vi "Butterfly_PullUp VPI VRL with Capacitance 20220628.vi"(0 "Semiconductor Module Context":T2, 3 "C_TH_Delta":dbl=0.03 format="%#_13g", 4 "VNAs Measurement Parameters":T1, 5 "error in (no error)":errorcluster, 9 "Start_v":dbl=10.0 format="%#_13g", 11 "Stop_v":dbl=41.0 format="%#_13g") -> (14 "Semiconductor Module Context Out":T2, 19 "error out":errorcluster)   [LabVIEW 2013]
uses:
  <vilib>/NI_TestStand_SemiconductorModule/NI_TestStand_Semiconductor_Module.lvlibp/PinMap/General/SemiconductorModuleContext.ctl
  VNA/VNAs Measurement Parameters.ctl
  <instrlib>/niDCPower/nidcpower.llb/niDCPower Wait For Event - Event.ctl
  <vilib>/NI_TestStand_SemiconductorModule/NI_TestStand_Semiconductor_Module.lvlibp/PinMap/General/Publish/PublishDataDouble2D.vi
  <vilib>/NI_TestStand_SemiconductorModule/NI_TestStand_Semiconductor_Module.lvlibp
  VNA/Pin Map API/VNA Custom Instrument.lvlib
panel:
  out "Site":i32
  out "RL Step":i32
  out "PI Step":i32
  out "C_TH_PU":dbl format="%#_3g"
  out "C_Free":dbl[](array[numeric]) format="%#_3g"
  out "max index":i32
  out "BF C PI":dbl format="%#_3g"
  out "C_VPI":dbl
  out "BF C RL":dbl format="%#_3g"
  out "C_VRL":dbl
  out "appended array":dbl[][](array[numeric]) format="%#_3g"
  out "S3 steps":dbl[](array[numeric]) format="%#_3g"
  out "S2 steps":dbl[](array[numeric]) format="%#_3g"
  out "S1 steps":dbl[](array[numeric]) format="%#_3g"
  out "S0 steps":dbl[](array[numeric]) format="%#_3g"
  out "BF values":dbl[](array[numeric])
  out "VRLs":dbl[](array[numeric])
  out "VPIs":dbl[](array[numeric])
  out "Multisite Cap Data":dbl[][][](array[numeric])
  out "BF Names":string[](array[string])
  out "BFSamples":i32
  in  "Step_v":dbl=1.0
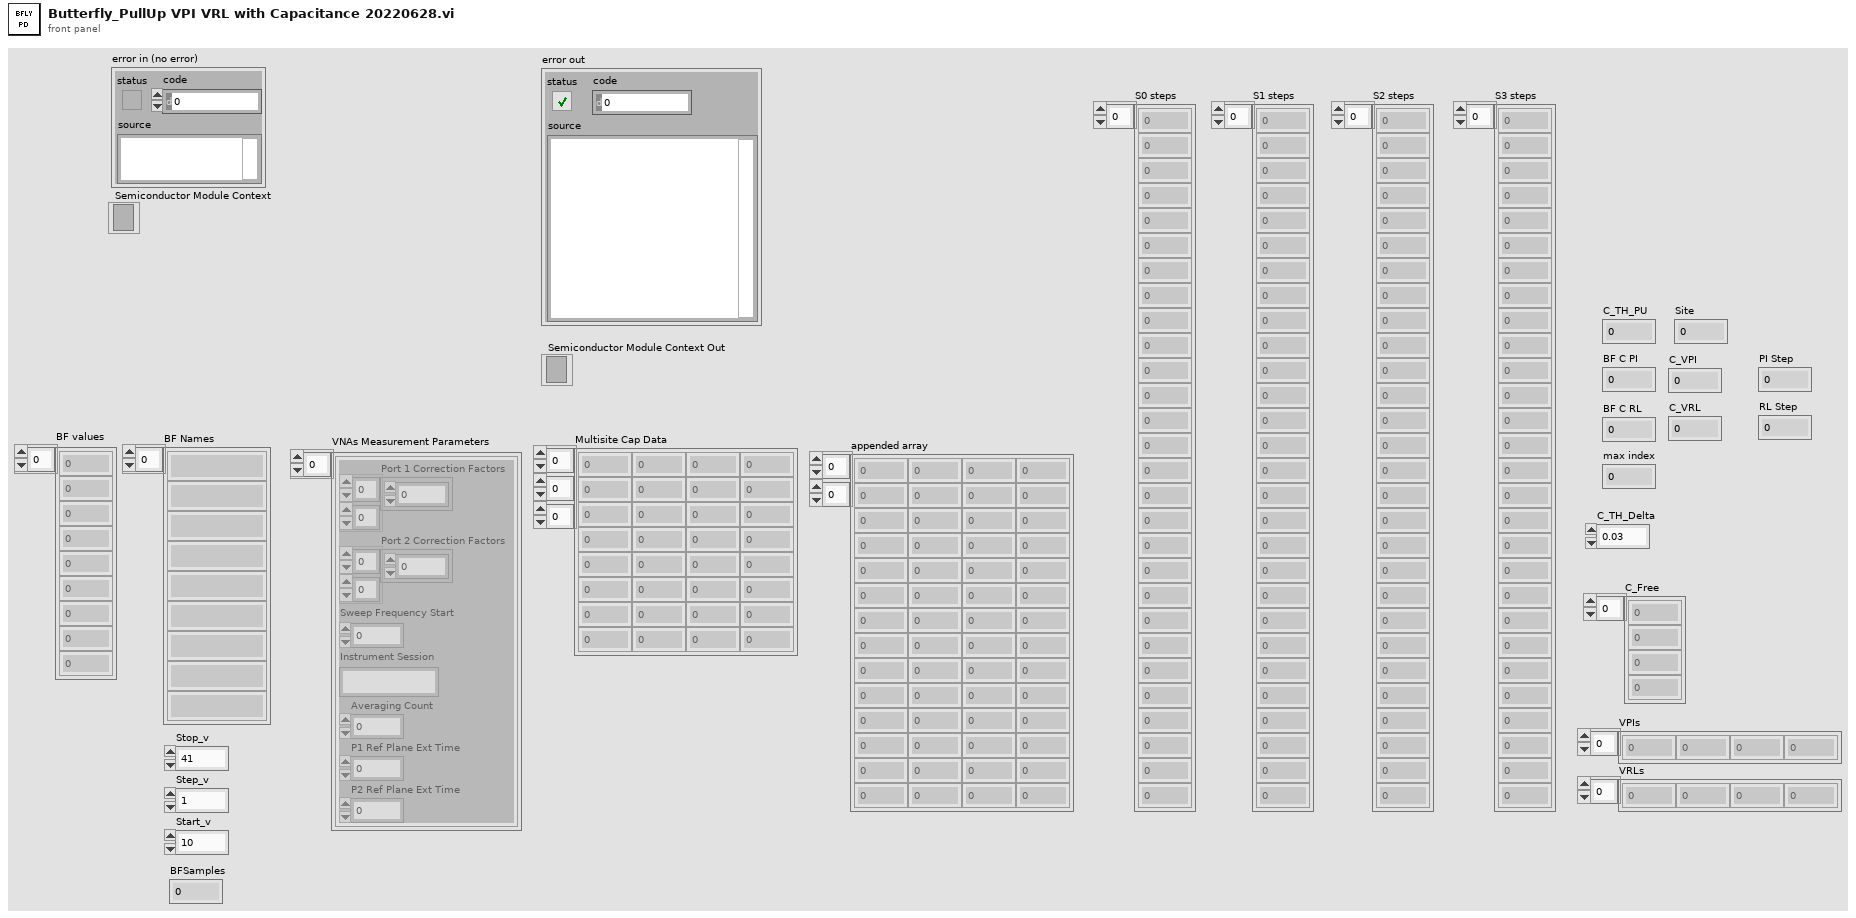
[diagram p1: front panel]
types:
  T1 = typedef "VNAs Measurement Parameters.ctl" = cluster{"Port 1 Correction Factors":cdb[][], "Port 2 Correction Factors":cdb[][], "Sweep Frequency Start":dbl, "Instrument Session":string, "Averaging Count":i32, "P1 Ref Plane Ext Time":dbl, "P2 Ref Plane Ext Time":dbl}[]
  T2 = typedef "NI_TestStand_Semiconductor_Module.lvlibp/SemiconductorModuleContext.ctl" = refnum<k7>
  T3 = typedef "niDCPower Wait For Event - Event.ctl" = i32
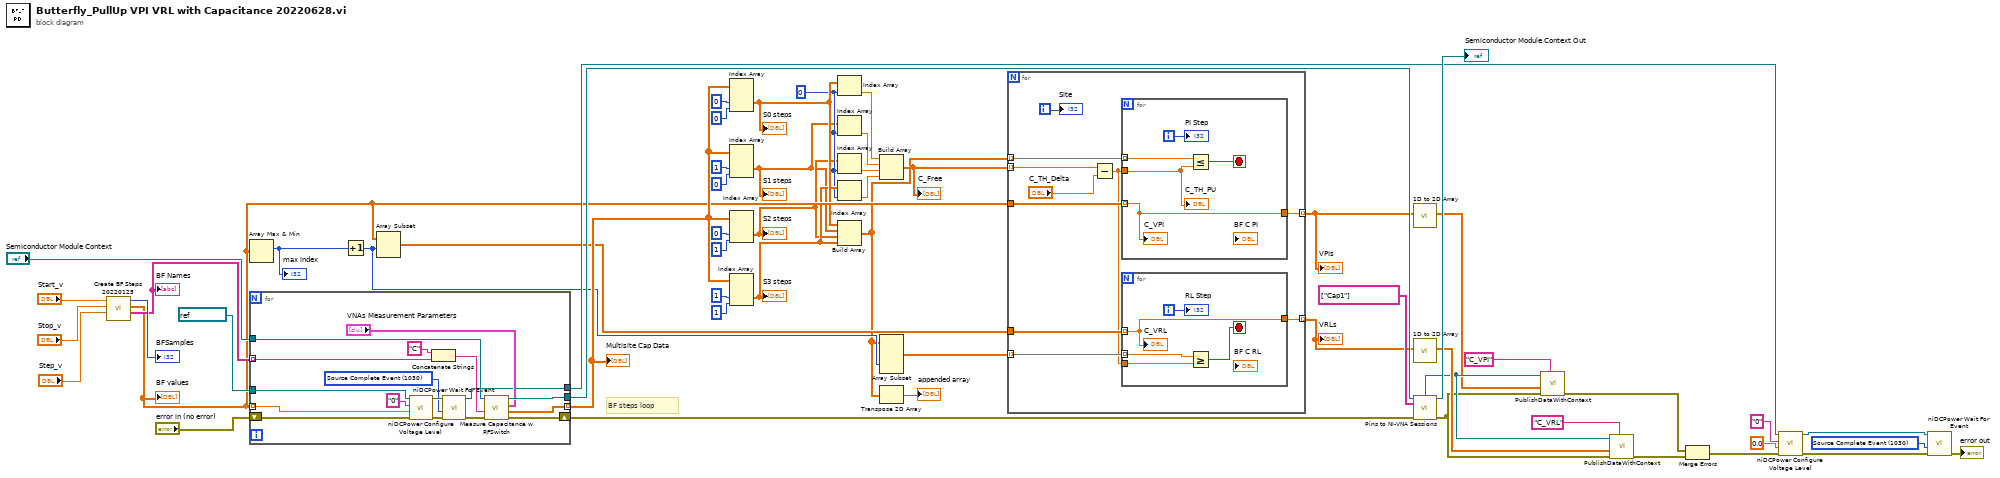
[diagram p0: block diagram]
diagram:
  w8 = 0 ("index")
  w40 = T3 1030 items=["Source Complete Event"=1030, "Measure Complete Event"=1031, "Sequence Iteration Complete Event"=1032, "Sequence Engine Done Event"=1033, "Pulse Complete Event"=1051, "Ready For Pulse Trigger Event"=1052] ("event")
  # "BF steps loop"
  n1 = call "Create BF Steps 20220125.vi"("Step_v"="Step_v", "Stop_v"="Stop_v", "Start_v"="Start_v") -> ("BF Names"=w49:string[], "BF values"=w15:dbl[], "BFSamples"=→"BFSamples":i32)  [unwired: 6 in]
  "BF Names" <- w49
  "BF values" <- w15
  n2 = Array Max & Min(array=w15) -> (max index (indices)=w17:i32)  [unwired: 3 out]
  "max index" <- w17
  n3 = for {
    shift-right: [w60] -> w38
    shift-left: "error in (no error)" -> [w64]
    tunnel: "Semiconductor Module Context" -> [w58]
    tunnel: [w73] -> w54
    tunnel: [w69] -> w39 mode=indexing
    tunnel: w49 -> [w68] mode=indexing
    tunnel: w15 -> [w63] mode=indexing
    tunnel: refnum<k15> "4139_1" ("instrument handle") -> [w62]
    tunnel: [w61] -> w44
    w66 = T3 1030 items=["Source Complete Event"=1030, "Measure Complete Event"=1031, "Sequence Iteration Complete Event"=1032, "Sequence Engine Done Event"=1033, "Pulse Complete Event"=1051, "Ready For Pulse Trigger Event"=1052] ("event")
    n4 = call <instrlib>:"niDCPower Configure Voltage Level.vi"("error in (no error)"=w64, "voltage level"=w63, "channel name"="0", "instrument handle"=w62) -> ("error out"=w65:errorcluster, "instrument handle out"=w67:refnum<k15>)  [unwired: 6 in]
    n5 = Concatenate Strings("C" ("string"), w68) -> (w71:string)
    n6 = call <instrlib>:"niDCPower Wait For Event.vi"("error in (no error)"=w65, "event"=w66, "instrument handle"=w67) -> ("error out"=w59:errorcluster, "instrument handle out"=w61:refnum<k15>)  [unwired: 7 in]
    n7 = call "Measure Capacitance w RFSwitch.vi"("VNAs Measurement Parameters"="VNAs Measurement Parameters", "error in (no error)"=w59, "Measurement Id"=w71, "Semiconductor Module Context"=w58) -> ("error out"=w60:errorcluster, "Multisite Cap Data"=w69:dbl[][], "Semiconductor Module Context Out"=w73:T2)  [unwired: 5 in]
  }
  "Multisite Cap Data" <- w39
  n8 = Increment(x=w17) -> (x+1=w16:i32)
  n9 = Array Subset(array=w15, index=w16) -> (w14:dbl[])  [unwired: 1 in]
  n10 = Index Array(array=w39, index (dim 1)=0 ("disabled index (row)"), index (dim 2)=0 ("disabled index (col)")) -> (element=w11:dbl[])  [unwired: 1 in]
  "S0 steps" <- w11
  n11 = Index Array(array=w39, index (dim 1)=1 ("index (row)"), index (dim 2)=0 ("index (col)")) -> (element=w2:dbl[])  [unwired: 1 in]
  "S1 steps" <- w2
  n12 = Index Array(array=w39, index (dim 1)=0 ("index (row)"), index (dim 2)=1 ("index (col)")) -> (element=w3:dbl[])  [unwired: 1 in]
  "S2 steps" <- w3
  n13 = Index Array(array=w39, index (dim 1)=1 ("index (row)"), index (dim 2)=1 ("index (col)")) -> (element=w9:dbl[])  [unwired: 1 in]
  "S3 steps" <- w9
  n14 = Index Array(array=w11, index=w8) -> (element=w10:dbl)
  n15 = Index Array(array=w2, index=w8) -> (element=w7:dbl)
  n16 = Index Array(array=w3, index=w8) -> (element=w5:dbl)
  n17 = Index Array(array=w9, index=w8) -> (element=w6:dbl)
  n18 = Build Array(w11, w2, w3, w9) -> (w1:dbl[][])
  n19 = Build Array(w10, w7, w5, w6) -> (w4:dbl[])
  "C_Free" <- w4
  n20 = Array Subset(array=w1, index (col)=w16) -> (w18:dbl[][])  [unwired: 3 in]
  n21 = Transpose 2D Array(2D array=w1) -> (transposed array=→"appended array":dbl[][])
  n22 = for {
    tunnel: w15 -> [w83]
    tunnel: [w82] -> w13 mode=indexing
    tunnel: w14 -> [w81]
    tunnel: w18 -> [w80] mode=indexing
    tunnel: [w79] -> w12 mode=indexing
    tunnel: w4 -> [w76] mode=indexing
    tunnel: w1 -> [w77] mode=indexing
    i -> [w78]
    n23 = Subtract(x=w76, y="C_TH_Delta") -> (x-y=w74:dbl)
    n24 = for {
      tunnel: w83 -> [w92] mode=indexing
      tunnel: [w92] -> w82
      tunnel: w74 -> [w91]
      tunnel: w77 -> [w89] mode=indexing
      i -> [w90]
      stop <- w93 stop-if-true
      n25 = Less Or Equal?(x=w89, y=w91) -> (x <= y?=w93:bool)
      "C_VPI" <- w92
      "C_TH_PU" <- w91
      "PI Step" <- w90
    }
    n26 = for {
      tunnel: w81 -> [w87] mode=indexing
      tunnel: w80 -> [w84] mode=indexing
      tunnel: [w87] -> w79
      tunnel: w74 -> [w86]
      i -> [w85]
      stop <- w88 stop-if-true
      n27 = Greater Or Equal?(x=w84, y=w86) -> (x >= y?=w88:bool)
      "C_VRL" <- w87
      "RL Step" <- w85
    }
    "Site" <- w78
  }
  "VPIs" <- w13
  "VRLs" <- w12
  n28 = call "1D to 2D Array.vi"("1D Array"=w13) -> ("2D Array"=w22:dbl[][])  [unwired: 10 in]
  n29 = call "1D to 2D Array.vi"("1D Array"=w12) -> ("2D Array"=w35:dbl[][])  [unwired: 10 in]
  n30 = call "Pins to NI-VNA Sessions.vi"("Semiconductor Module Context"=w54, "Pins"=string[] ["Cap1"] ("Capacitance Pins"), "error in (no error)"=w38) -> ("Pin Query Context"=w23:refnum<class "MultiplePinMultipleSessionQueryContext.lvclass">, "Semiconductor Module Context Out"=→"Semiconductor Module Context Out":T2, "error out"=w19:errorcluster)  [unwired: 8 in, 2 out]
  n31 = call-poly <vilib>:"PublishDataWithContext.vi"("Published Data Id"="C_VPI", "error in (no error)"=w19, "Data In"=w22, "Pin Query Context"=w23) -> ("error out"=w20:errorcluster)  [unwired: 6 in, 1 out]
  n32 = call-poly <vilib>:"PublishDataWithContext.vi"("Published Data Id"="C_VRL", "error in (no error)"=w19, "Data In"=w35, "Pin Query Context"=w23) -> ("error out"=w36:errorcluster)  [unwired: 6 in, 1 out]
  n33 = Merge Errors(w20, w36) -> (w37:errorcluster)
  n34 = call <instrlib>:"niDCPower Configure Voltage Level.vi"("error in (no error)"=w37, "voltage level"=0.0, "channel name"="0", "instrument handle"=w44) -> ("error out"=w43:errorcluster, "instrument handle out"=w41:refnum<k15>)  [unwired: 6 in]
  n35 = call <instrlib>:"niDCPower Wait For Event.vi"("error in (no error)"=w43, "event"=w40, "instrument handle"=w41) -> ("error out"=→"error out":errorcluster)  [unwired: 7 in, 1 out]
